vi "Initial Parameters From Particle Data.vi"(9 "Particle Reports (Pixels)":T3(array[cluster]), 10 "Src Image":T1, 11 "Masked Image":T1) -> (3 "Array":T2(array[cluster]))   [LabVIEW 2011]
uses:
  <vilib>/vision/Image Controls.llb/IMAQ Image.ctl
  <vilib>/vision/NI_Vision_Development_Module.lvlib
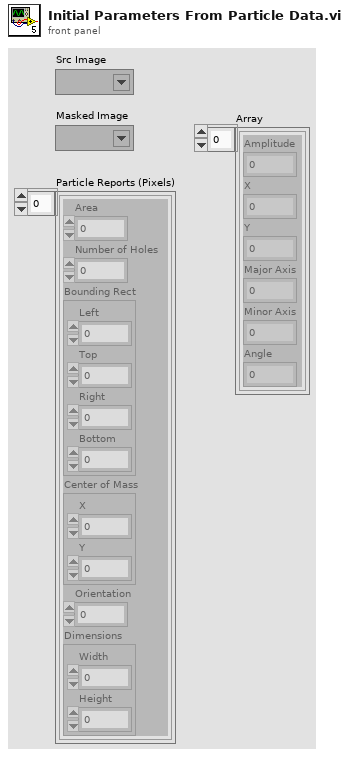
[diagram p1: front panel]
types:
  T1 = typedef "IMAQ Image.ctl" = refnum<image>
  T2 = cluster{"Amplitude":dbl, "X":dbl, "Y":dbl, "Major Axis":dbl, "Minor Axis":dbl, "Angle":dbl}[]
  T3 = cluster{"Area":dbl, "Number of Holes":dbl, "Bounding Rect":cluster{"Left":dbl, "Top":dbl, "Right":dbl, "Bottom":dbl}, "Center of Mass":cluster{"X":dbl, "Y":dbl}, "Orientation":dbl, "Dimensions":cluster{"Width":dbl, "Height":dbl}}[]
  T4 = cluster{"Amplitude":dbl, "X":dbl, "Y":dbl, "Major Axis":dbl, "Minor Axis":dbl, "Angle":dbl}
  T5 = typedef "Particle Parameters" = i32
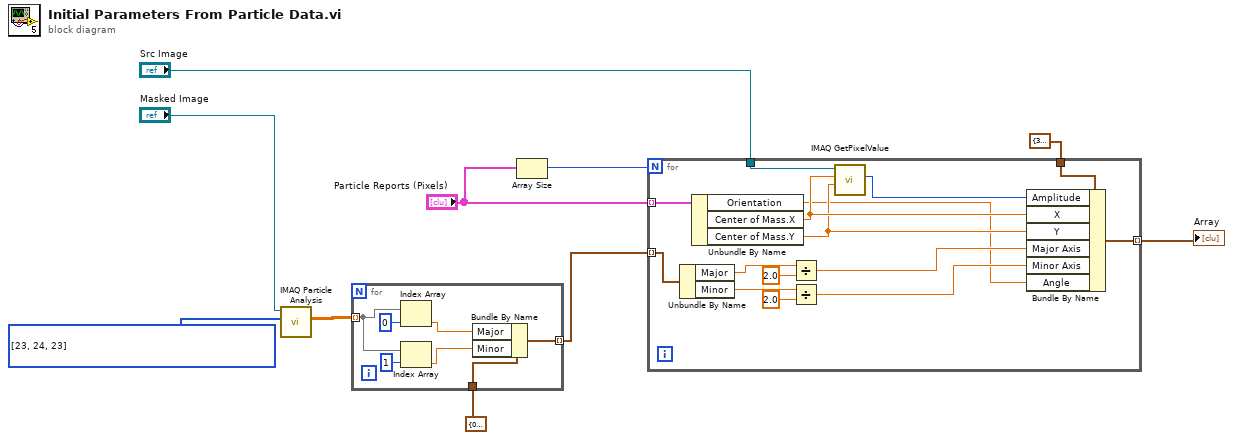
[diagram p0: block diagram]
diagram:
  w9 = T5[] [23, 24, 23] items=["Center of Mass X", "Center of Mass Y", "First Pixel X", "First Pixel Y", "Bounding Rect Left", "Bounding Rect Top", "Bounding Rect Right", "Bounding Rect Bottom", "Max Feret Diameter Start X", "Max Feret Diameter Start Y", "Max Feret Diameter End X", "Max Feret Diameter End Y", "Max Horiz. Segment Length Left", "Max Horiz. Segment Length Right", "Max Horiz. Segment Length Row", "-", "Bounding Rect Width", "Bounding Rect Height", "Bounding Rect Diagonal", "Perimeter", "Convex Hull Perimeter", "Holes' Perimeter", "Max Feret Diameter", "Equivalent Ellipse Major Axis", "Equivalent Ellipse Minor Axis", "Equivalent Ellipse Minor Axis (Feret)", "Equivalent Rect Long Side", "Equivalent Rect Short Side", "Equivalent Rect Diagonal", "Equivalent Rect Short Side (Feret)", "Average Horiz. Segment Length", "Average Vert. Segment Length", "Hydraulic Radius", "Waddel Disk Diameter", "-", "Area", "Holes' Area", "Particle & Holes' Area", "Convex Hull Area", "Image Area", "-", "Number of Holes", "Number of Horiz. Segments", "Number of Vert. Segments", "-", "Orientation", "Max Feret Diameter Orientation", "-", "% Area/Image Area", "% Area/(Particle & Holes' Area)", "Ratio of Equivalent Ellipse Axes", "Ratio of Equivalent Rect Sides", "-", "Elongation Factor", "Compactness Factor", "Heywood Circularity Factor", "Type Factor", "-", "Sum X", "Sum Y", "Sum XX", "Sum XY", "Sum YY", "Sum XXX", "Sum XXY", "Sum XYY", "Sum YYY", "-", "Moment of Inertia XX", "Moment of Inertia XY", "Moment of Inertia YY", "Moment of Inertia XXX", "Moment of Inertia XXY", "Moment of Inertia XYY", "Moment of Inertia YYY", "Norm. Moment of Inertia XX", "Norm. Moment of Inertia XY", "Norm. Moment of Inertia YY", "Norm. Moment of Inertia XXX", "Norm. Moment of Inertia XXY", "Norm. Moment of Inertia XYY", "Norm. Moment of Inertia YYY", "Hu Moment 1", "Hu Moment 2", "Hu Moment 3", "Hu Moment 4", "Hu Moment 5", "Hu Moment 6", "Hu Moment 7"] ("Pixel Measurements")
  n1 = call "IMAQ Particle Analysis"("Pixel Measurements"=w9, "Image"="Masked Image") -> ("Particle Measurements (Pixels)"=w8:dbl[][])  [unwired: 4 in, 5 out]
  n2 = for {
    tunnel: w8 -> [w16] mode=indexing
    tunnel: cluster{"Major":dbl, "Minor":dbl} {"Major"=0.0, "Minor"=0.0} ("Ellipse Axes") -> [w17]
    tunnel: [w11] -> w5 mode=indexing
    n3 = Index Array(array=w16, index=0) -> (element=w13:dbl)
    n4 = Index Array(array=w16, index=1) -> (element=w12:dbl)
    n5 = Bundle By Name(cluster=w17, "Major"=w13, "Minor"=w12) -> (w11:cluster{"Major":dbl, "Minor":dbl})
  }
  n6 = Array Size(array="Particle Reports (Pixels)") -> (size(s)=w2:i32)
  n7 = for {
    N: w2 -> [_]
    tunnel: "Particle Reports (Pixels)" -> [w32] mode=indexing
    tunnel: w5 -> [w30] mode=indexing
    tunnel: "Src Image" -> [w31]
    tunnel: T4 {"Amplitude"=372.03255698316156, "X"=8.089344924052103, "Y"=15.142360409795089, "Major Axis"=14.647769362592497, "Minor Axis"=8.289444397456732, "Angle"=80.06042857407111} -> [w25]
    tunnel: [w18] -> w3 mode=indexing
    n8 = Unbundle By Name(w30) -> ("Major"=w29:dbl, "Minor"=w28:dbl)
    n9 = Unbundle By Name(w32) -> ("Orientation"=w20:dbl, "Center of Mass.X"=w24:dbl, "Center of Mass.Y"=w23:dbl)
    n10 = Divide(x=w29, y=2.0) -> (x/y=w22:dbl)
    n11 = Divide(x=w28, y=2.0) -> (x/y=w21:dbl)
    n12 = call "IMAQ GetPixelValue"("Image"=w31, "X Coordinate"=w24, "Y Coordinate"=w23) -> ("Pixel Value (I16)"=w19:i16)  [unwired: 3 in, 4 out]
    n13 = Bundle By Name(cluster=w25, "Amplitude"=w19, "X"=w24, "Y"=w23, "Major Axis"=w22, "Minor Axis"=w21, "Angle"=w20) -> (w18:T4)
  }
  "Array" <- w3
